vi "dereference string pointer.vi"(8 "error in":errorcluster, 10 "data buffer":u64, 11 "count":i32) -> (0 "error out":errorcluster, 3 "byte array":u8[](array[numeric]))   [LabVIEW 2013, in "lvnano.lvlib"]
uses:
  lvnano.lvlib
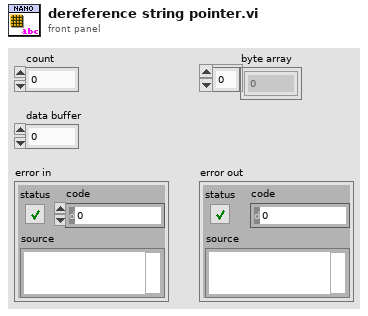
[diagram p1: front panel]
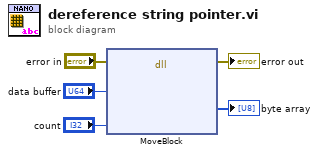
[diagram p0: block diagram]
diagram:
  n1 = dll-call lib="LabVIEW" fn="MoveBlock"(error in="error in", "source pointer"="data buffer", "count"="count") -> (error out=→"error out":errorcluster, "destination pointer"=→"byte array":u8[])  [unwired: 6 in, 1 out]
